vi "Robot Main.vi"() -> ()   [LabVIEW 2016]
doc: "This VI implements the framework and scheduler for your robotics program. It should not be necessary to modify the framework. You are expected to add your code to the VIs called from Robot Main - the ones located in the Team Code folder within the project."
uses:
  <vilib>/Rock Robotics/WPI/ThirdParty/CanMotor/TalonSRX/WPI_CANTalonSRX_APIControlMode.ctl
  <vilib>/Rock Robotics/WPI/ThirdParty/CanMotor/TalonSRX/WPI_CANTalonSRX_BrakeOverride.ctl
  <vilib>/Rock Robotics/SystemInterfaces/DIO/FPGA_DIOChannel.ctl
  <vilib>/Rock Robotics/WPI/SafetyOutput/WPI_SafetyOutputConfigMenu.ctl
  <vilib>/Platform/TimedLoop/XDataNode/timing_clust.ctl
  <vilib>/Platform/TimedLoop/XDataNode/nitl_modes.ctl
  <vilib>/Platform/TimedLoop/XDataNode/wakeup.ctl
  <vilib>/Rock Robotics/WPI/Counter/WPI_CounterDigitalInputToDigitalSource.vi
  <vilib>/Rock Robotics/WPI/Counter/WPI_CounterOpen Semi Period Mode.vi
  <vilib>/addons/control/pid/pid.llb/PID (DBL).vi
  <vilib>/platform/TimedLoop/XDataNode/XDataNode.xnode
  <vilib>/Platform/TimedLoop/XDataNode/XDNodeRunTimeDep.lvlib
  <vilib>/addons/control/pid/NI_PID_pid.lvlib
panel:
  in  "Invert":bool
  in  "Device Number":u8
  in  "Control Mode":T1
  in  "Brake / Coast Mode":T2=enum."Override to Coast"
  in  "timeout (s)":dbl=0.1
  in  "Loop Period us":i64=1000
  in  "output range":cluster{"output high":dbl, "output low":dbl}={"output high"=0.4, "output low"=0.0} {"output low" format="%.2f"; "output high" format="%.2f"}
  in  "PID gains":T3={"proportional gain (Kc)"=0.0018, "integral time (Ti, min)"=0.0, "derivative time (Td, min)"=0.0} {"derivative time (Td, min)" format="%.3f"; "integral time (Ti, min)" format="%.3f"; "proportional gain (Kc)" format="%.4f"}
  in  "Speed Target":dbl=0.00025 format="%#_13g"
  in  "FF Gain":dbl=0.000216 format="%#_13g"
  in  "sample length":i32=512
  out "RPM":dbl=2312.02290444024
  in  "Counter Factor":dbl=60.0 format="%#_13g"
  out "Stopped":bool
  in  "Number Samples to Average":u8=1 min=1 max=128
  in  "stop":bool
  in  "High Pulse (T)":bool
  in  "Digital Pin":T4=enum."DIO 1"
  out "Waveform Chart":cluster{dbl, "Speed Target":dbl}(graph)
  out "error out":errorcluster
  in  "error in":errorcluster
  # "<-- (1/encoder period) * (counter factor) = RPM"
  # "counter factor = (1/1024) * 60\n\n1024 since semi period mode only \nmeasures duration of low pulse? or 1/512 \nsince it measures from one low pulse to the next?"
  # "for 512 PPR:\n0.05859375"
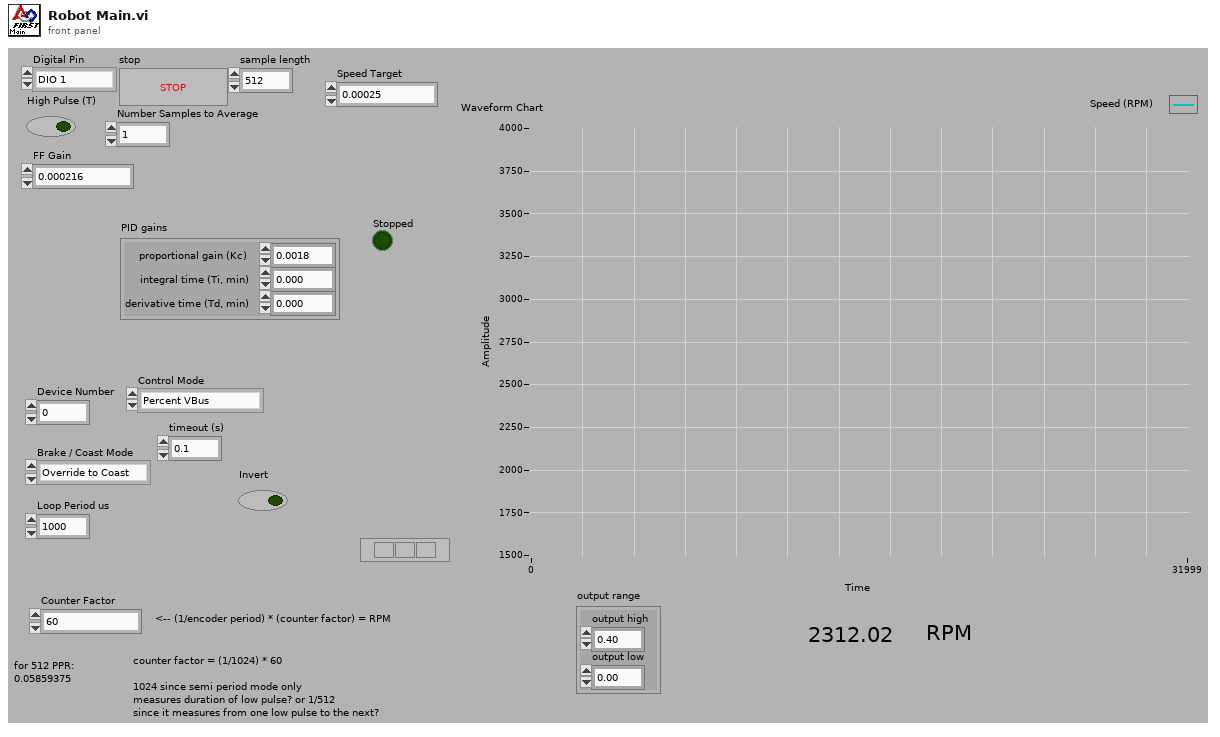
[diagram p1: front panel]
types:
  T1 = typedef "WPI_CANTalonSRX_APIControlMode.ctl" = enum8{"Percent VBus", "Speed", "Position", "Slave", "Unchanged / Invalid", "Voltage Compensation", "Current", "Motion Profile", "Motion Magic"}
  T2 = typedef "WPI_CANTalonSRX_BrakeOverride.ctl" = enum8{"No Override", "Override to Coast", "Override to Brake"}
  T3 = cluster{"proportional gain (Kc)":dbl, "integral time (Ti, min)":dbl, "derivative time (Td, min)":dbl}
  T4 = typedef "FPGA_DIOChannel.ctl" = enum8{"DIO 0", "DIO 1", "DIO 2", "DIO 3", "DIO 4", "DIO 5", "DIO 6", "DIO 7", "DIO 8", "DIO 9", "DIO MXP 0", "DIO MXP 1", "DIO MXP 2", "DIO MXP 3", "DIO MXP 4", "DIO MXP 5", "DIO MXP 6", "DIO MXP 7", "DIO MXP 8", "DIO MXP 9", "DIO MXP 10", "DIO MXP 11", "DIO MXP 12", "DIO MXP 13", "DIO MXP 14", "DIO MXP 15", "SPI Port CS1", "SPI Port CS2", "SPI Port CS3", "SPI Port MISO", "SPI Port MOSI", "Invalid"}
  T5 = typedef "WPI_SafetyOutputConfigMenu.ctl" = enum16{"Enable", "Disable"}
  T6 = typedef "WPI_DigitalInputDevRef.ctl" = cluster{"DevStatus":errorcluster, "DIO Channel":T4}
  T7 = typedef "FPGA_CounterEncoderSourceConvertionLVSourceType.ctl" = cluster{"DevStatus":errorcluster, "AnalogTriggerMode?":bool, "DigitalMode":cluster{"DIO Channel":T8}, "AnalogTriggerMode":cluster{"AnalogTriggerIndex":T9, "OutputType":T10}}
  T8 = typedef "FPGA_DIODigitalSourceChannel.ctl" = enum8{"DIO 0", "DIO 1", "DIO 2", "DIO 3", "DIO 4", "DIO 5", "DIO 6", "DIO 7", "DIO 8", "DIO 9", "DIO MXP 0", "DIO MXP 1", "DIO MXP 2", "DIO MXP 3", "DIO MXP 4", "DIO MXP 5", "DIO MXP 6", "DIO MXP 7", "DIO MXP 8", "DIO MXP 9", "DIO MXP 10", "DIO MXP 11", "DIO MXP 12", "DIO MXP 13", "DIO MXP 14", "DIO MXP 15", "Disabled"}
  T9 = typedef "FPGA_AnalogTriggerIndex.ctl" = enum8{"Trig 0", "Trig 1", "Trig 2", "Trig 3", "Trig 4", "Trig 5", "Trig 6", "Trig 7", "Invalid"}
  T10 = typedef "FPGA_AnalogTriggerOutType.ctl" = enum16{"InWindow", "TriggerState", "Rising", "Falling"}
  T11 = typedef "WPI_MotorControlDeviceRef.ctl" = cluster{"DeviceStatus":errorcluster, "Type":T12, "PWM":cluster{"PWM Channel":T13, "DeadBand":T14}, "CAN":cluster{"Device Number":u8, "SetOutput VI Ref":variant, "GetOutput VI Ref":variant, "Enable VI Ref":variant, "Disable VI Ref":variant, "Data":variant}, "Invert":bool}
  T12 = typedef "WPI_MotorControlType.ctl" = enum16{"PWM", "CAN"}
  T13 = typedef "FPGA_DIOPWMChannel.ctl" = enum8{"PWM 0", "PWM 1", "PWM 2", "PWM 3", "PWM 4", "PWM 5", "PWM 6", "PWM 7", "PWM 8", "PWM 9", "PWM MXP 0", "PWM MXP 1", "PWM MXP 2", "PWM MXP 3", "PWM MXP 4", "PWM MXP 5", "PWM MXP 6", "PWM MXP 7", "PWM MXP 8", "PWM MXP 9", "Invalid"}
  T14 = typedef "WPI_PWMDeadband.ctl" = cluster{"Name":string, "maxPositivePwm":i32, "minPositivePwm":i32, "centerPwm":i32, "maxNegativePwm":i32, "minNegativePwm":i32, "angularRange":u16}
  T15 = typedef "WPI_CounterDevRef.ctl" = cluster{"DevStatus":errorcluster, "CntIndex":T16}
  T16 = typedef "FPGA_CounterCtrSystemIndex.ctl" = enum8{"Ctr 0", "Ctr 1", "Ctr 2", "Ctr 3", "Ctr 4", "Ctr 5", "Ctr 6", "Ctr 7", "Invalid"}
  T17 = typedef "XDNodeRunTimeDep.lvlib/timing_clust.ctl" = cluster{"Expected End [f-1]":u64, "Actual End [f-1]":u64, "Finished Late? [f-1]":bool, "Expected End [i-1]":u64, "Actual End [i-1]":u64, "Finished Late? [i-1]":bool, "Expected Start [i]":u64, "Actual Start [i]":u64, "Expected Start [f]":u64, "Actual Start [f]":u64, "Source Name":string, "Structure Name":string, "Period":i64, "Deadline":i64, "Offset":i64, "Start":i64, "Priority":i32, "Timeout":i32, "Mode":T18, "Wakeup Reason":T19, "Error":errorcluster, "Source Type":string, "Secondary Source Type":string, "Global End Time":u64, "Global Start Time":u64, "Frame Duration":u64, "Iteration Duration":u64, "Assigned CPU":i32, "I/O Scan Engine Mode":u32}
  T18 = typedef "XDNodeRunTimeDep.lvlib/nitl_modes.ctl" = enum32{"No Change", "Process missed periods, maintain original phase", "Discard missed periods, maintain original phase", "Process missed periods, ignore original phase", "Discard missed periods, ignore original phase"}
  T19 = typedef "XDNodeRunTimeDep.lvlib/wakeup.ctl" = enum32{"Normal", "Aborted", "Asynchronous wakeup", "Timing source error", "Timed loop error", "Timeout"}
  T20 = cluster{"MotorControlDevRef":T11, "CounterDevRef out":T15}
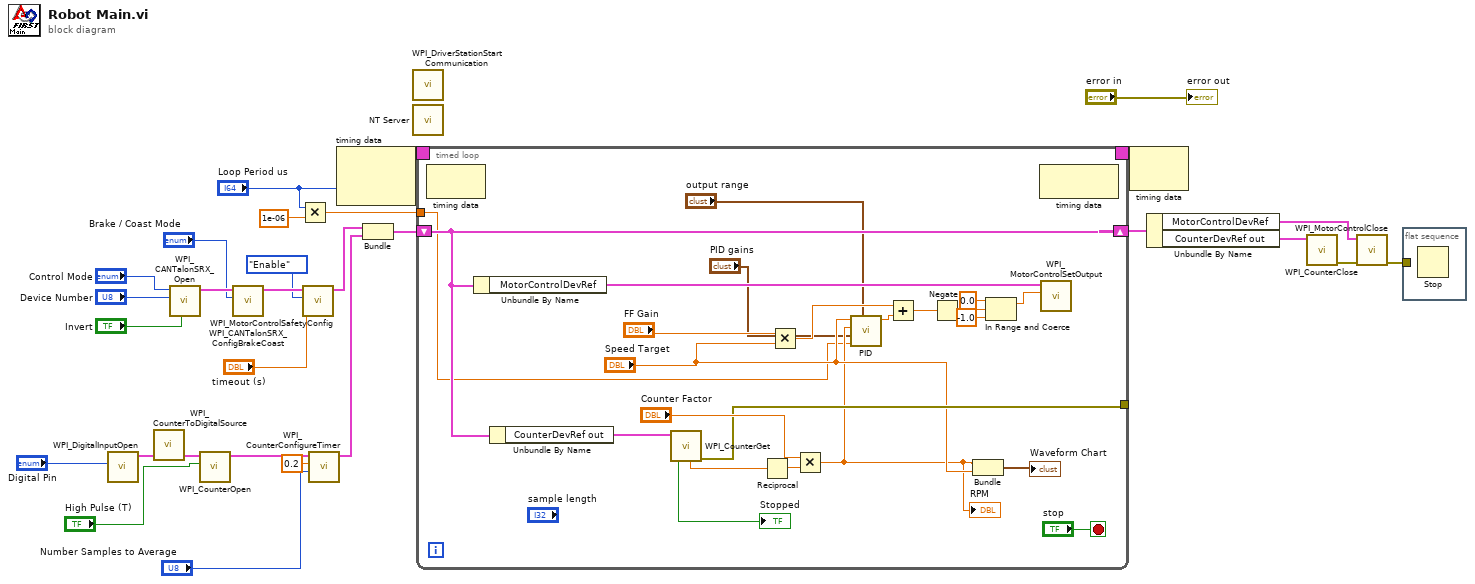
[diagram p0: block diagram]
diagram:
  n1 = call <vilib>:"WPI_DigitalInputOpen.vi"("DIO Channel"="Digital Pin") -> ("DigitalInputDevRef"=w16:T6)  [unwired: 1 in, 9 out]
  n2 = call-poly <vilib>:"WPI_CounterToDigitalSource.vi"("DigitalInputDevRef"=w16) -> ("Digital Source"=w18:T7)  [unwired: 6 out]
  n3 = call <vilib>:"WPI_CANTalonSRX_Open.vi"("Invert"="Invert", "Device Number"="Device Number", "Control Mode"="Control Mode") -> ("CAN Talon SRX Ref"=w26:T11)  [unwired: 7 in, 1 out]
  n4 = call-poly <vilib>:"WPI_CounterOpen.vi"("High Pulse (T)"="High Pulse (T)", "Source"=w18) -> ("CounterDevRef"=w14:T15)  [unwired: 3 in, 6 out]
  n5 = call <vilib>:"WPI_CANTalonSRX_ConfigBrakeCoast.vi"("Brake / Coast Mode"="Brake / Coast Mode", "CAN Talon SRX Ref"=w26) -> ("CAN Talon SRX Ref"=w24:T11)  [unwired: 8 in, 1 out]
  n6 = Multiply(x="Loop Period us", y=1e-06 ("upper limit")) -> (x*y=w1:dbl)
  n7 = call <vilib>:"WPI_MotorControlSafetyConfig.vi"("timeout (s)"="timeout (s)", "mode"=WPI_SafetyOutputConfigMenu."Enable", "MotorControlDevRef"=w24) -> ("MotorControlDevRef"=w19:T11)  [unwired: 7 in, 1 out]
  n8 = call <vilib>:"WPI_CounterConfigureTimer.vi"("Number Samples to Average"="Number Samples to Average", "MaxPeriod (sec)"=0.2, "CounterDevRef in"=w14) -> ("CounterDevRef out"=w12:T15)  [unwired: 7 in, 1 out]
  n9 = node-c288("Loop Period us") -> (w21:T17)  [unwired: 1 in]
  n10 = Bundle("MotorControlDevRef"=w19, "CounterDevRef out"=w12) -> (w13:T20)  [unwired: 1 in]
  n11 = call <vilib>:"WPI_DriverStationStart Communication.vi"() -> ()  [unwired: 2 in, 10 out]
  n12 = call <vilib>:"NT Server.vi"() -> ()  [unwired: 12 in]
  n13 = timed-loop {
    timing: w21 -> [_]
    timing-out: [_] -> w20
    shift-right: [w51] -> w8
    shift-left: w13 -> [w51]
    tunnel: [w45] -> _
    tunnel: w1 -> [w30]
    stop <- "stop" stop-if-true
    n14 = node-c288() -> ()  [unwired: 1 in, 1 out]
    n15 = Unbundle By Name(w51) -> ("MotorControlDevRef"=w44:T11)
    n16 = Unbundle By Name(w51) -> ("CounterDevRef out"=w50:T15)
    n17 = call <vilib>:"WPI_CounterGet.vi"("CounterDevRef in"=w50) -> ("error out"=w45:errorcluster, "Period (sec)"=w48:dbl, "Stopped"=→"Stopped":bool)  [unwired: 5 in, 3 out]
    n18 = Reciprocal(x=w48) -> (1/x=w47:dbl)
    n19 = Multiply(x="FF Gain", y="Speed Target") -> (x*y=w41:dbl)
    n20 = Multiply(x="Counter Factor", y=w47) -> (x*y=w38:dbl)
    "RPM" <- w38
    n21 = call-poly <vilib>:"PID.vi"("output range"="output range", "dt (s)"=w30, "PID gains"="PID gains", "process variable"=w38, "setpoint"="Speed Target") -> ("output"=w35:dbl)  [unwired: 5 in, 1 out]
    n22 = Add(x=w41, y=w35) -> (x+y=w40:dbl)
    n23 = Negate(x=w40) -> (-x=w34:dbl)
    n24 = Bundle(w38, "Speed Target"="Speed Target") -> (→"Waveform Chart":cluster{dbl, "Speed Target":dbl})  [unwired: 1 in]
    n25 = In Range and Coerce(upper limit=0.0, x=w34, lower limit=-1.0) -> (coerced(x)=w33:dbl)  [unwired: 1 out]
    n26 = node-c288() -> ()  [unwired: 1 in, 1 out]
    n27 = call <vilib>:"WPI_MotorControlSetOutput.vi"("Output"=w33, "MotorControlDevRef"=w44) -> ()  [unwired: 7 in, 3 out]
  }
  n28 = node-c288(w20) -> ()  [unwired: 1 out]
  n29 = Unbundle By Name(w8) -> ("MotorControlDevRef"=w7:T11, "CounterDevRef out"=w6:T15)
  n30 = call <vilib>:"WPI_CounterClose.vi"("CounterDevRef"=w6) -> ("error out"=w5:errorcluster)  [unwired: 10 in]
  n31 = call <vilib>:"WPI_MotorControlClose.vi"("error in"=w5, "MotorControlDevRef"=w7) -> ("error out"=w4:errorcluster)  [unwired: 9 in]
  n32 = flat-sequence {
    tunnel: w4 -> [_]
    frame #0 {
      n33 = Stop() -> ()  [unwired: 1 in]
    }
  }
  "error out" <- "error in"
